vi "Read ALRP.vi"(8 "error in (no error)":errorcluster, 11 "Alarms in":T4) -> (0 "error out":errorcluster, 2 "ALRP":T1, 3 "Alarms out":T4)   [LabVIEW 2019, in "Alarms.lvlib"]
uses:
  Alarms.lvlib
  Ctl/Alarms.ctl
  Ctl/ALR_defs.ctl
  Ctl/ALRs_State.ctl
  Ctl/ALR_ON_OFF.ctl
  Ctl/ALR_Parameters.ctl
  Ctl/ALR code.ctl
  Ctl/ALR type.ctl
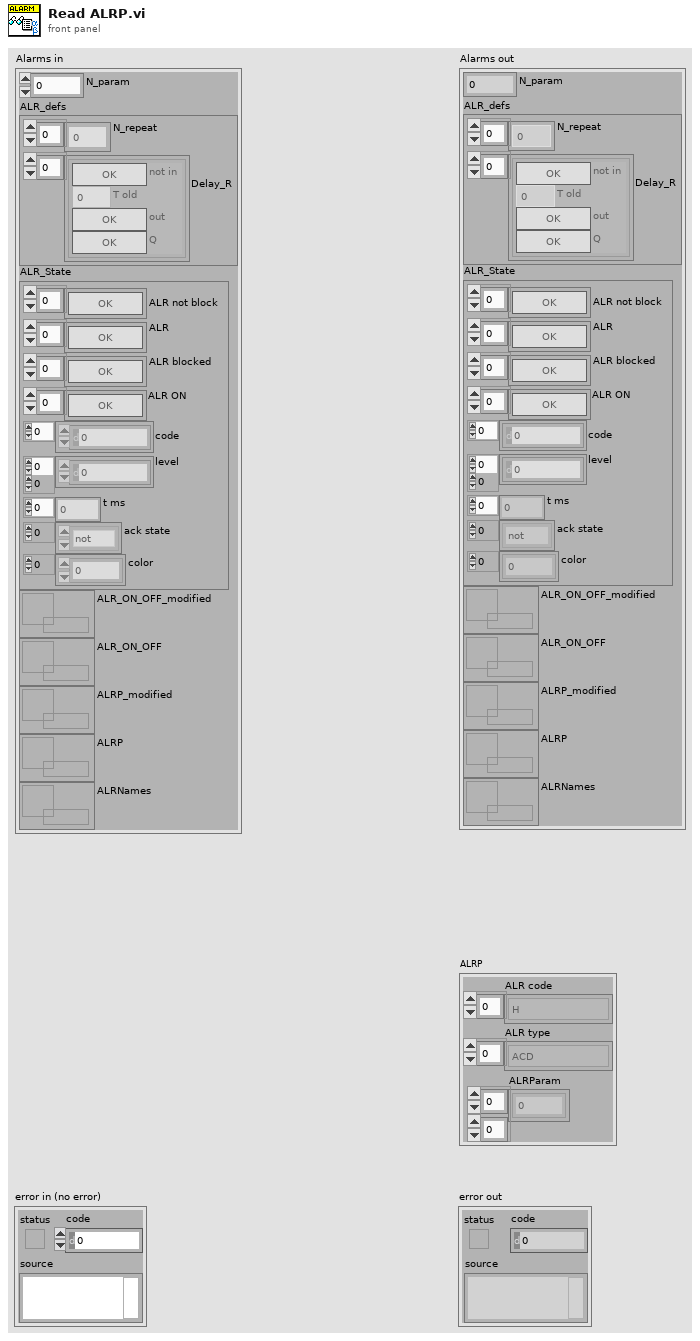
[diagram p1: front panel]
types:
  T1 = typedef "Alarms.lvlib/ALR_Parameters.ctl" = cluster{"ALR code":T2[], "ALR type":T3[], "ALRParam":u32[][]}
  T2 = typedef "Alarms.lvlib/ALR code.ctl" = enum16{"CONN", "H", "HH", "L", "LL", "SERR", "ON", "OFF", "XM19", "XM24", "XM47", "XM51", "XM52", "XM53", "XM54", "XM55", "XM56", "XM61", "XM62", "XM63", "XM64", "XM65", "XM66"}
  T3 = typedef "Alarms.lvlib/ALR type.ctl" = enum16{"ACD", "ACDR", "ALRN", "ALR"}
  T4 = typedef "Alarms.lvlib/Alarms.ctl" = cluster{"N_param":i32, "ALR_defs":T5, "ALR_State":T6, "ALR_ON_OFF_modified":refnum<data-value>, "ALR_ON_OFF":refnum<data-value>, "ALRP_modified":refnum<data-value>, "ALRP":refnum<data-value>, "ALRNames":refnum<data-value>}
  T5 = typedef "Alarms.lvlib/ALR_defs.ctl" = cluster{"N_repeat":u32[], "Delay_R":cluster{"not in":bool, "T old":u32, "out":bool, "Q":bool}[]}
  T6 = typedef "Alarms.lvlib/ALRs_State.ctl" = cluster{"ALR not block":bool[], "ALR":bool[], "ALR blocked":bool[], "ALR ON":bool[], "code":i32[], "level":i32[][], "t ms":u32[], "ack state":enum32{"not", "tripped", "reset", "ack"}[], "color":u32[]}
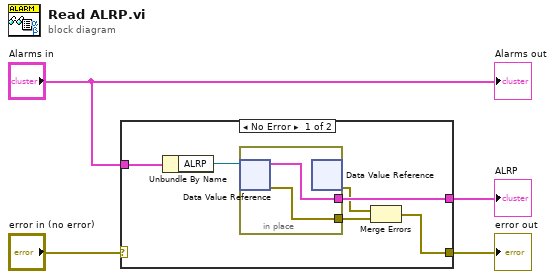
[diagram p0: block diagram]
diagram:
  n1 = case shown="No Error" "error in (no error)" {
    selector: "error in (no error)" -> [_ w13]
    tunnel: [w6 w13] -> w3
    tunnel: "Alarms in" -> [w5 _]
    tunnel: [w9 _] -> w2
    frame No Error {
      n2 = Unbundle By Name(w5) -> ("ALRP"=w10:refnum<data-value>)
      n3 = in-place {
        in-place-border: [w12] -> w8
        in-place-border: [w11] -> w9
        n4 = in-place-dvr #1(w10) -> (w11:T1, w12:errorcluster)
        n5 = in-place-dvr #1() -> (w7:errorcluster)  [unwired: 1 in, 1 out]
      }
      n6 = Merge Errors(w7, w8) -> (w6:errorcluster)
    }
    frame Error {
    }
  }
  "error out" <- w3
  "ALRP" <- w2
  "Alarms out" <- "Alarms in"
